vi "Auto Locate.vi"(1 "Autonomous?":bool) -> (0 "X Drive Arcade":dbl)   [LabVIEW 2012]
uses:
  BotStatus.vi
  Motors Values.vi
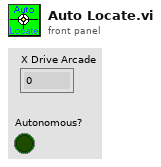
[diagram p1: front panel]
types:
  T1 = cluster{"Target Position X":dbl, "Target Position Y":dbl, "Target Found":bool}
  T2 = typedef "WPI_ServoDeviceRef.ctl" = cluster{"DeviceStatus":errorcluster, "Digital Module":T3, "PWM Channel":T4, "DeadBand":T5}
  T3 = typedef "FPGA_TypedefDigitalModule.ctl" = enum16{"Digital Module 1", "Digital Module 2"}
  T4 = typedef "FPGA_DIOPWMChannel.ctl" = enum8{"PWM 1", "PWM 2", "PWM 3", "PWM 4", "PWM 5", "PWM 6", "PWM 7", "PWM 8", "PWM 9", "PWM 10", "Invalid"}
  T5 = typedef "WPI_PWMDeadband.ctl" = cluster{"Name":string, "maxPositivePwm":i32, "minPositivePwm":i32, "centerPwm":i32, "maxNegativePwm":i32, "minNegativePwm":i32, "angularRange":u16}
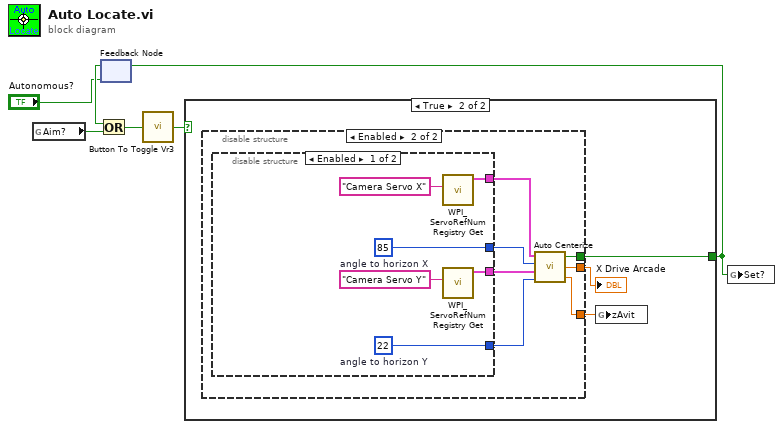
[diagram p0: block diagram]
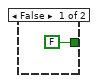
[diagram p2: hidden frame]
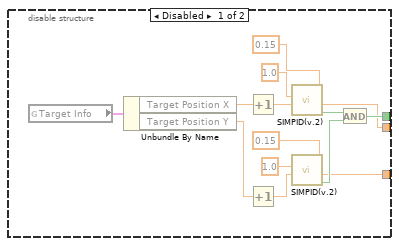
[diagram p3: hidden frame]
diagram:
  n1 = global read "BotStatus.vi" "Aim?"() -> (w3:bool)
  n2 = feedback #1("Autonomous?") -> (w2:bool)
  n3 = Or(x=w2, y=w3) -> (x .or. y?=w4:bool)
  n4 = call "Button To Toggle Vr3.vi"("InValue"=w4) -> ("Result"=w6:bool)
  n5 = case shown="True" w6 {
    tunnel: [FALSE w10] -> w5
    frame False {
    }
    frame True {
      n6 = disable-structure shown="Enabled" {
        disable-tunnel: [w13 w27] -> w10
        disable-tunnel: [w12 w26] -> w9
        disable-tunnel: [w11 w25] -> w8
        frame Disabled {
          n7 = global read "BotStatus.vi" "Target Info"() -> (w24:T1)
          n8 = Unbundle By Name(w24) -> ("Target Position X"=w19:dbl, "Target Position Y"=w23:dbl)
          n9 = Increment(x=w19) -> (x+1=w18:dbl)
          n10 = Increment(x=w23) -> (x+1=w22:dbl)
          n11 = call "SIMPID(v.2).vi"("Range"=0.15, "Current Point"=w18, "Set Point"=1.0) -> ("On Target"=w14:bool, "result"=w12:dbl)  [unwired: 7 in]
          n12 = call "SIMPID(v.2).vi"("Range"=0.15, "Current Point"=w22, "Set Point"=1.0) -> ("On Target"=w15:bool, "result"=w11:dbl)  [unwired: 7 in]
          n13 = And(x=w14, y=w15) -> (x .and. y?=w13:bool)
        }
        frame Enabled {
          n14 = disable-structure shown="Enabled" {
            disable-tunnel: [w36 _] -> w31
            disable-tunnel: [w34 _] -> w30
            disable-tunnel: [w33 _] -> w29
            disable-tunnel: [w32 _] -> w28
            frame Enabled {
              w32 = u16 22  # angle to horizon Y
              w33 = u16 85  # angle to horizon X
              n15 = call <vilib>:"WPI_ServoRefNum Registry Get.vi"("refnum name"="Camera Servo X") -> ("ServoDeviceRef"=w36:T2)  [unwired: 9 in, 1 out]
              n16 = call <vilib>:"WPI_ServoRefNum Registry Get.vi"("refnum name"="Camera Servo Y") -> ("ServoDeviceRef"=w34:T2)  [unwired: 9 in, 1 out]
            }
            frame Disabled {
            }
          }
          n17 = call "Auto Centerize.vi"("angle to horizon Y"=w28, "Camera Y ServoDeviceRef"=w30, "angle to horizon X"=w29, "Camera X ServoDeviceRef"=w31) -> ("zAvit"=w25:dbl, "X Drive Arcade"=w26:dbl, "Centerized?"=w27:bool)
        }
      }
      "X Drive Arcade" <- w9
      n18 = global write "Motors Values.vi" "zAvit"(w8) -> ()
    }
  }
  n19 = feedback-in #1(w5) -> ()
  n20 = global write "BotStatus.vi" "Set?"(w5) -> ()
